vi "PH_IEEE1394Camera.State On.vi"(0 "VI in":refnum<vi>, 2 "IMAQ1394 Session in":T1, 5 "error in (no error)":errorcluster) -> (14 "VI out":refnum<vi>, 16 "IMAQ1394 Session out":T1, 18 "Cam Error":errorcluster, 19 "error out":errorcluster)   [LabVIEW 2014, in "PH_IEEE1394Camera.lvlib"]
uses:
  PH_IEEE1394Camera.lvlib
  <vilib>/userdefined/High Color/IMAQdx.ctl
  <vilib>/vision/driver/NI_Vision_Acquisition_Software.lvlib
  PH_Cam_BaseClass/PH_Cam_BaseClass.lvlib
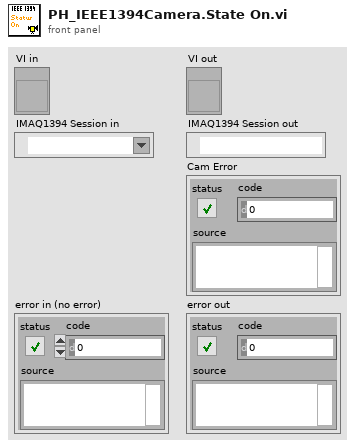
[diagram p1: front panel]
types:
  T1 = typedef "IMAQdx.ctl" = refnum<k21>
  T2 = typedef "PH_Cam_BaseClass.lvlib/PH_Cam_BaseClass.i attribute.ctl" = cluster{"Gui Refs":T3, "Cam":cluster{"Source Notifier":refnum<notifier>, "Error":errorcluster, "Camera ID":string}, "Images":cluster{"Cam":T4, "Operation":T4, "PSDB":T4}, "Window Image":cluster{"Indicate Image":bool, "Window No.":i32, "Scale Facor":dbl, "Center Cross":bool, "Subtract Backgr":bool, "CoG":bool, "Color Palette":cluster{"Red":u8, "Green":u8, "Blue":u8}[], "Image On":bool}, "Default Prdc Int":i32, "Performance":cluster{"on":bool, "Timestamp Last Frame":i32}, "Histogram":cluster{"on":bool, "Mapping":bool}, "Save Image":cluster{"Save":bool, "File refnum":refnum<file>}, "Setting Service ID":i32, "Screen":cluster{"x-resolution":i16, "y-resolution":i16}, "On":bool, "Constructor finished":bool, "configured":bool}
  T3 = typedef "PH_Cam_BaseClass.lvlib/PH_Cam_BaseClass.GUI Refs.ctl" = cluster{"Frame Rate":refnum<vi>, "Get Frame Rate":refnum<vi>, "Show Image":refnum<vi>, "Get Histogram":refnum<vi>, "Mapping":refnum<vi>, "Histogram":refnum<vi>, "Center Cross":refnum<vi>, "Center of Gravity":refnum<vi>, "Scale Factor [%]":refnum<vi>, "Save Image":refnum<vi>, "Palette":refnum<vi>, "Subtract Background":refnum<vi>, "Cam Error":refnum<vi>, "On":refnum<vi>, "Cam List":refnum<vi>}
  T4 = typedef "IMAQ Image.ctl" = refnum<image>
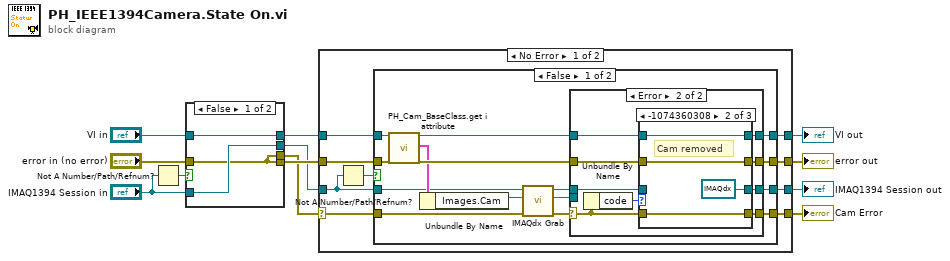
[diagram p0: block diagram]
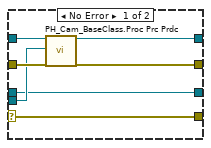
[diagram p2: hidden frame]
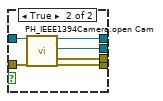
[diagram p7: hidden frame]
diagram:
  n1 = Not A Number/Path/Refnum?(number/path/refnum="IMAQ1394 Session in") -> (NaN/Path/Refnum?=w6:bool)
  n2 = case shown="False" w6 {
    tunnel: "VI in" -> [w14 w21]
    tunnel: [w14 w20] -> w9
    tunnel: "error in (no error)" -> [w13 w19]
    tunnel: [w13 w18] -> w8
    tunnel: [w15 w17] -> w7
    tunnel: [w13 w16] -> w5
    tunnel: "IMAQ1394 Session in" -> [w15 _]
    frame False {
    }
    frame True {
      n3 = call "PH_IEEE1394Camera.open Cam.vi"("VI in"=w21, "error in (no error)"=w19) -> ("VI out"=w20:refnum<vi>, "Cam Session Out"=w17:T1, "Cam Error out"=w16:errorcluster, "error out"=w18:errorcluster)  [unwired: 14 in]
    }
  }
  n4 = case shown="No Error" w5 {
    selector: w5 -> [w27 w78]
    tunnel: [w30 w78] -> w12
    tunnel: [w29 w79] -> w11
    tunnel: [w28 w80] -> w10
    tunnel: w9 -> [w26 w80]
    tunnel: w8 -> [w25 w79]
    tunnel: w7 -> [w23 w77]
    tunnel: [w22 w77] -> w1
    frame No Error {
      n5 = Not A Number/Path/Refnum?(number/path/refnum=w23) -> (NaN/Path/Refnum?=w24:bool)
      n6 = case shown="False" w24 {
        tunnel: [w45 w74] -> w30
        tunnel: [w44 w75] -> w29
        tunnel: [w43 w76] -> w28
        tunnel: w23 -> [w34 w73]
        tunnel: w27 -> [w33 w74]
        tunnel: w26 -> [w40 w76]
        tunnel: w25 -> [w38 w75]
        tunnel: [w31 w73] -> w22
        frame False {
          n7 = call "PH_Cam_BaseClass.get i attribute.vi"("i ref in"=w40, "error in (no error)"=w38) -> ("i ref out"=w39:refnum<vi>, "i attribute"=w36:T2, "error out"=w37:errorcluster)  [unwired: 15 in]
          n8 = Unbundle By Name(w36) -> ("Images.Cam"=w35:T4)
          n9 = call <vilib>:"IMAQdx Grab.vi"("error in"=w33, "Image In"=w35, "Session In"=w34) -> ("error out"=w42:errorcluster, "Image Out"=w41:T4, "Session Out"=w32:T1)  [unwired: 5 in, 1 out]
          n10 = case shown="Error" w42 {
            selector: w42 -> [w48 w55]
            tunnel: w39 -> [w52 w60]
            tunnel: w41 -> [w47 _]
            tunnel: [w50 w61] -> w44
            tunnel: w37 -> [w49 w57]
            tunnel: [w51 w59] -> w43
            tunnel: [w48 w56] -> w45
            tunnel: w32 -> [w46 w54]
            tunnel: [w46 w53] -> w31
            frame No Error {
              n11 = call "PH_Cam_BaseClass.Proc Prc Prdc.vi"("VI in"=w52, "Image In"=w47, "error in (no error)"=w49) -> ("VI out"=w51:refnum<vi>, "error out"=w50:errorcluster)  [unwired: 15 in]
            }
            frame Error {
              n12 = Unbundle By Name(w55) -> ("code"=w58:i32)
              n13 = case shown="-1074360308" w58 {
                tunnel: [w63 w67 w71] -> w61
                tunnel: w60 -> [w64 w68 w72]
                tunnel: [w64 w68 w72] -> w59
                tunnel: w57 -> [w63 w67 w71]
                tunnel: [w63 w65 w70] -> w56
                tunnel: w55 -> [_ w65 w70]
                tunnel: w54 -> [w62 _ w69]
                tunnel: [w62 T1 refnum ("Session Out") w69] -> w53
                frame -1074360293 {
                  # "Timeout"
                }
                frame -1074360308 {
                  # "Cam removed"
                }
                frame Default {
                }
              }
            }
          }
        }
        frame True {
        }
      }
    }
    frame Error {
    }
  }
  "Cam Error" <- w12
  "error out" <- w11
  "VI out" <- w10
  "IMAQ1394 Session out" <- w1
